vi "Maya2000 - get a spectrum + wavelengths.vi"(8 "error in (no error)":errorcluster, 10 "This instrments index":i32, 11 ".NET Refnum in":refnum<k24>) -> (0 "error out":errorcluster, 1 "Wavelengths":dbl[](array[numeric]), 2 "Spectrum":dbl[](array[numeric]), 3 ".NET Refnum out":refnum<k24>, 4 "Is saturated?":bool, 5 "Start, end time one sepctrum":timestamp[](array[timestamp]))   [LabVIEW 2016]
doc: "Gets the spectrum and wavelengths array from one UV spectrometer.\nAdded support for start and end time. Not sure it is useful and correct wrt. the delta\ntime as the spectrometer may be free-running at programmed rate.\nThere is a built in timer which could be used."
uses:
  C:/Program Files/Ocean Optics/OmniDriver/OOI_HOME/NETOmniDriver-NET40.dll
  Program Files/Ocean Optics/OmniDriver/OOI_HOME/NETOmniDriver-NET40.dll
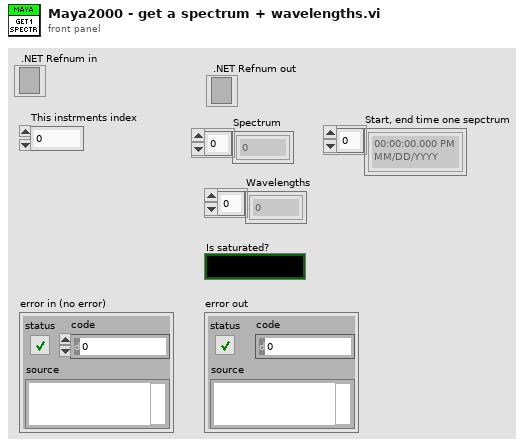
[diagram p1: front panel]
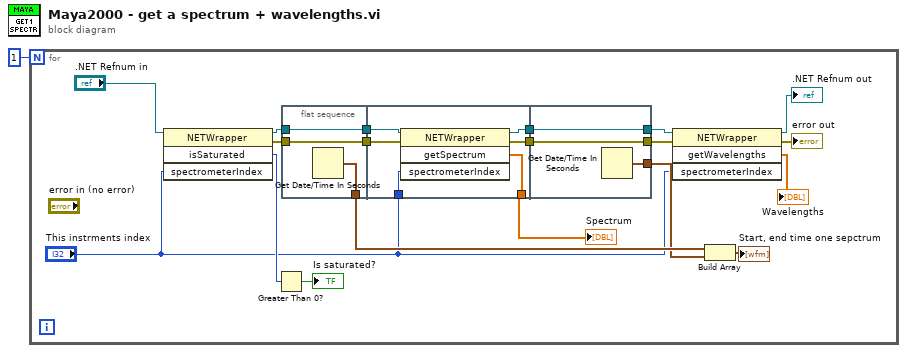
[diagram p0: block diagram]
diagram:
  n1 = for {
    N: 1 -> [_]
    n2 = invoke class="NETWrapper" method="isSaturated"(reference=".NET Refnum in", "spectrometerIndex"="This instrments index") -> (reference out=w11:refnum<k24>, error out=w10:errorcluster, "isSaturated"=w15:i16)  [unwired: 2 in, 1 out]
    n3 = Greater Than 0?(x=w15) -> (x > 0?=→"Is saturated?":bool)
    n4 = flat-sequence {
      tunnel: w11 -> [w22]
      tunnel: w10 -> [w21]
      tunnel: [w21] -> w20
      tunnel: [w22] -> w19
      tunnel: [w23] -> w6
      tunnel: w20 -> [w27]
      tunnel: w19 -> [w28]
      tunnel: [w24] -> w7
      tunnel: "This instrments index" -> [w29]
      tunnel: [w26] -> w18
      tunnel: [w25] -> w17
      tunnel: [w30] -> w8
      tunnel: [w31] -> w9
      tunnel: [w32] -> w5
      tunnel: w18 -> [w30]
      tunnel: w17 -> [w31]
      frame #0 {
        n5 = Get Date/Time In Seconds() -> (seconds since 1Jan1904=w23:timestamp)
      }
      frame #1 {
        n6 = invoke class="NETWrapper" method="getSpectrum"(reference=w28, error in=w27, "spectrometerIndex"=w29) -> (reference out=w26:refnum<k24>, error out=w25:errorcluster, "getSpectrum"=w24:dbl[])  [unwired: 1 in, 1 out]
      }
      frame #2 {
        n7 = Get Date/Time In Seconds() -> (seconds since 1Jan1904=w32:timestamp)
      }
    }
    n8 = invoke class="NETWrapper" method="getWavelengths"(reference=w8, error in=w9, "spectrometerIndex"="This instrments index") -> (reference out=→".NET Refnum out":refnum<k24>, error out=→"error out":errorcluster, "getWavelengths"=→"Wavelengths":dbl[])  [unwired: 1 in, 1 out]
    n9 = Build Array(w6, w5) -> (→"Start, end time one sepctrum":timestamp[])
    "Spectrum" <- w7
  }
